vi "adjacent_ttl_parameters.vi"(8 "Deprivation\nparameters":T1={"Frame Row"=0, "Kstd"=40.0, "# Images for\nsleep detection"=10, "Kmean"=1.5, "Start time of sleep detection (images):"=1000, 0, "Length (images)"=3600, "# TTL"=10000, "by x images after first detection"=0, "PauseBetween TTL pulses"=0, "\nby x detections"=9, "# Total immobility\n detections"=0.0, "Pause max # adjacent\nTTL"=0.0, "TTL x start\ntime deprivation\n"=0.0, "Max #\nadjacent TTL"=10000, " Ca2+\nmode"=0} {"?" items=["1", "2", "3", "4"]; "Frame Row" items=["1", "2", "3", "4"]}, 10 "Input \nparameters":T3={"Frame rate (ms)"=2000, "Worm strain"="N2", "Time t"=0, "State"=enum."Image acquisition", "Time elapsed"=0.0, "Max_num_runs"=100000, "#TTL"=0, "Time of start TTL"=100000, "ImSub Value"=0, "Time of last TTL"=0, "Number of Columns"=2, "Number of Rows"=2, "# Adjacent TTL"=0, "Sleep deprivation status"="", "Sleep Detection"=FALSE, "# Sleep detections"=0, "Time of first sleep detection"=0, "Time max # adjacent TTL"=0, "Image t-1"=[], "Image t"=[]} {"Number of Rows" items=["1"=1, "2"=2, "3"=3, "4"=4]; "Number of Columns" items=["1"=1, "2"=2, "3"=3, "4"=4]}) -> (2 "Output \nparameters":T4={"Frame rate (ms)"=2000, "Worm strain"="N2", "Time t"=0, "State"=enum."Image acquisition", "Time elapsed"=0.0, "Max_num_runs"=100000, "#TTL"=0, "Time of start TTL"=100000, "ImSub Value"=0, "Time of last TTL"=0, "Number of Columns"=2, "Number of Rows"=2, "# AdjacentTTL"=0, "Sleep deprivation status"="", "Sleep Detection"=FALSE, "# Sleep detections"=0, "Time of first sleep detection"=0, "Time max # adjacent TTL"=0, "Image t-1"=[], "Image t"=[]} {"Number of Rows" items=["1"=1, "2"=2, "3"=3, "4"=4]; "Number of Columns" items=["1"=1, "2"=2, "3"=3, "4"=4]})   [LabVIEW 2011]
uses:
  state.ctl
panel:
  # "Sleep deprivation settings"
  # "Select deprivation animal"
  # "Row"
  # "Column"
  # "Sleep detection parameters"
  # "Sleep deprivation parameters"
  # "Delay deprivation start:"
  # "Pause deprivation (images):"
  # "Stop deprivation after:"
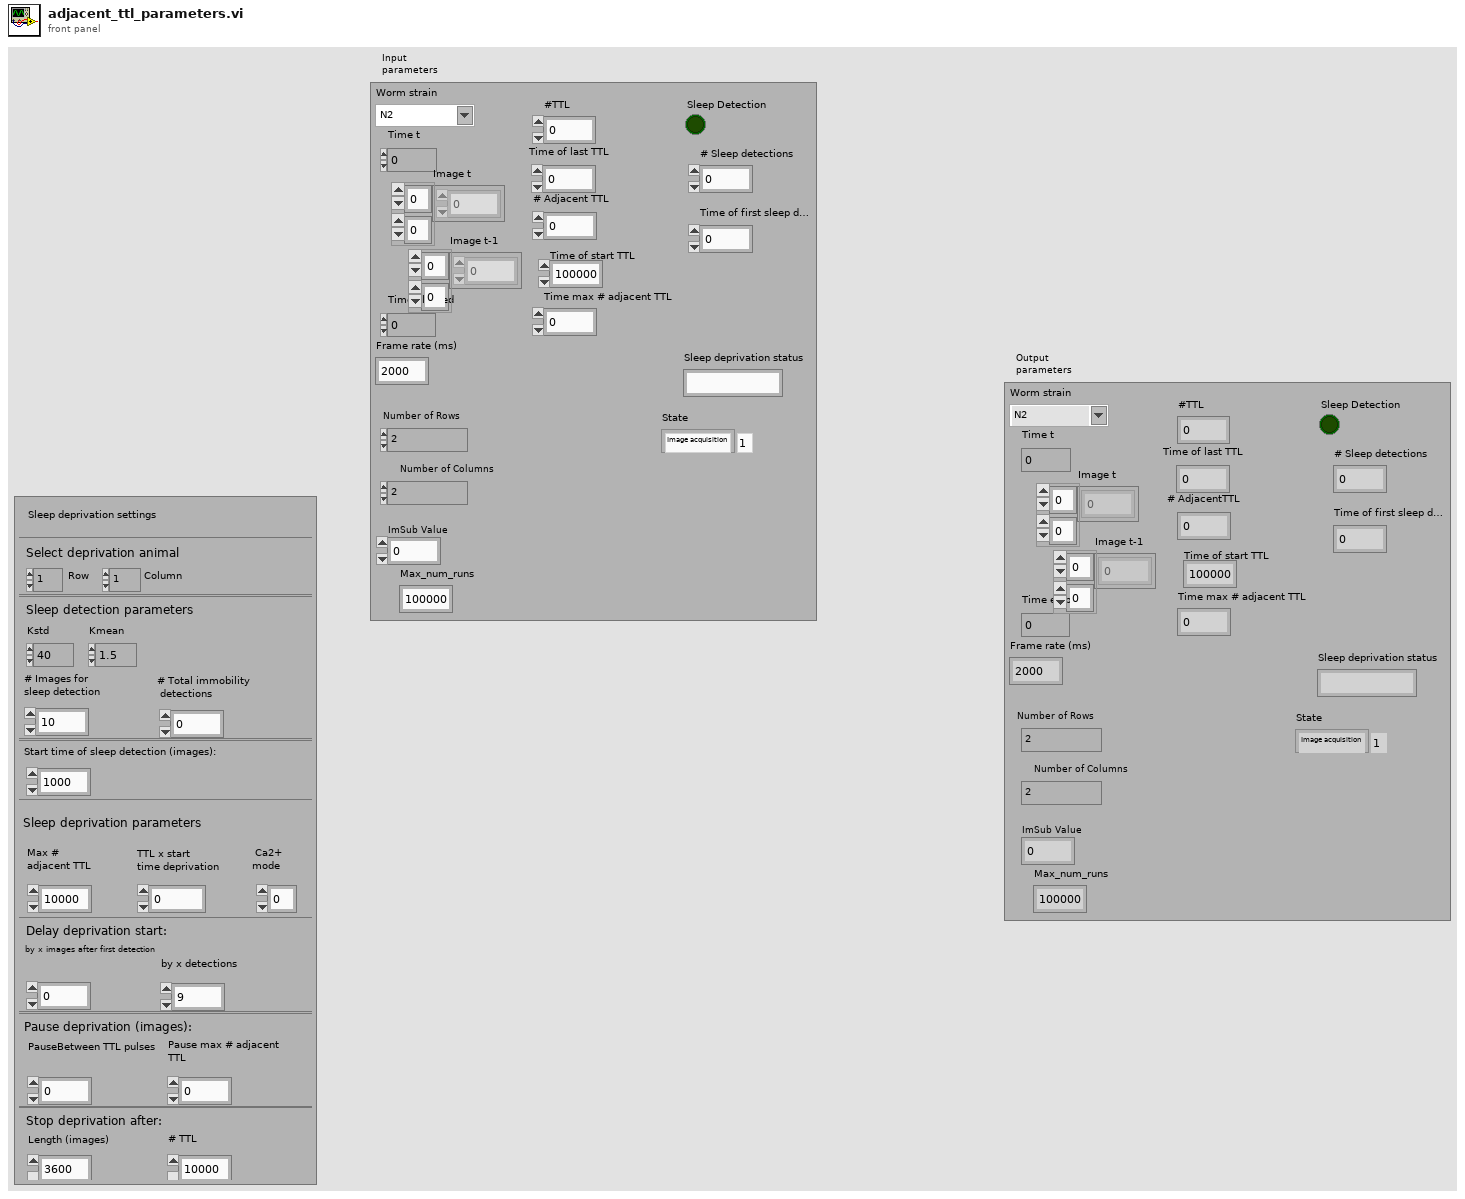
[diagram p1: front panel]
types:
  T1 = cluster{"Frame Row":u32, "Kstd":dbl, "# Images for\nsleep detection":i32, "Kmean":dbl, "Start time of sleep detection (images):":i32, u32, "Length (images)":i32, "# TTL":i32, "by x images after first detection":i32, "PauseBetween TTL pulses":i32, "\nby x detections":i32, "# Total immobility\n detections":dbl, "Pause max # adjacent\nTTL":dbl, "TTL x start\ntime deprivation\n":dbl, "Max #\nadjacent TTL":i32, " Ca2+\nmode":i32}
  T2 = typedef "state.ctl" = enum16{"Initialize measurement", "Image acquisition", "Image processing", "Sleep detection", "Control TTL protocol ", "Sleep deprivation", "Update image & exit condition", "Wait "}
  T3 = cluster{"Frame rate (ms)":u32, "Worm strain":string, "Time t":i32, "State":T2, "Time elapsed":dbl, "Max_num_runs":i32, "#TTL":i32, "Time of start TTL":i32, "ImSub Value":i32, "Time of last TTL":i32, "Number of Columns":u32, "Number of Rows":u32, "# Adjacent TTL":i32, "Sleep deprivation status":string, "Sleep Detection":bool, "# Sleep detections":i32, "Time of first sleep detection":i32, "Time max # adjacent TTL":i32, "Image t-1":i32[][], "Image t":i32[][]}
  T4 = cluster{"Frame rate (ms)":u32, "Worm strain":string, "Time t":i32, "State":T2, "Time elapsed":dbl, "Max_num_runs":i32, "#TTL":i32, "Time of start TTL":i32, "ImSub Value":i32, "Time of last TTL":i32, "Number of Columns":u32, "Number of Rows":u32, "# AdjacentTTL":i32, "Sleep deprivation status":string, "Sleep Detection":bool, "# Sleep detections":i32, "Time of first sleep detection":i32, "Time max # adjacent TTL":i32, "Image t-1":i32[][], "Image t":i32[][]}
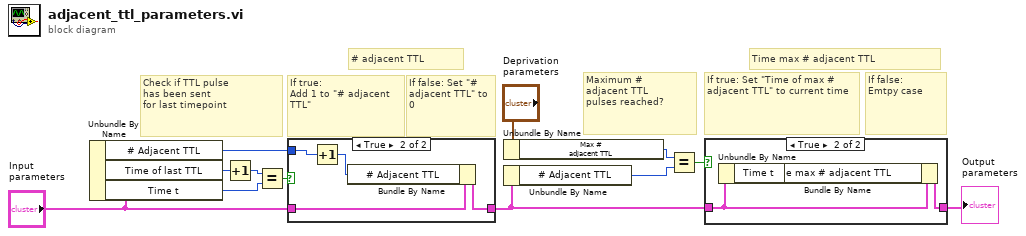
[diagram p0: block diagram]
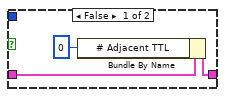
[diagram p2: hidden frame]
diagram:
  # "Maximum # \nadjacent TTL\npulses reached?"
  # "# adjacent TTL"
  # "Check if TTL pulse \nhas been sent \nfor last timepoint"
  # "If false: Set \"# adjacent TTL\" to 0"
  # "If true:\nAdd 1 to \"# adjacent TTL\""
  # "If false: \nEmtpy case"
  # "If true: Set \"Time of max # adjacent TTL\" to current time"
  # "Time max # adjacent TTL"
  n1 = Unbundle By Name("Input \nparameters") -> ("# Adjacent TTL"=w5:i32, "Time of last TTL"=w6:i32, "Time t"=w7:i32)
  n2 = Increment(x=w6) -> (x+1=w8:i32)
  n3 = Equal?(x=w8, y=w7) -> (x = y?=w9:bool)
  n4 = case shown="True" w9 {
    tunnel: "Input \nparameters" -> [w15 w18]
    tunnel: [w14 w19] -> w4
    tunnel: w5 -> [_ w16]
    frame False {
      n5 = Bundle By Name(cluster=w15, "# Adjacent TTL"=0 ("number of adjecentTTL")) -> (w14:T3)
    }
    frame True {
      n6 = Increment(x=w16) -> (x+1=w17:i32)
      n7 = Bundle By Name(cluster=w18, "# Adjacent TTL"=w17) -> (w19:T3)
    }
  }
  n8 = Unbundle By Name("Deprivation\nparameters") -> ("Max #\nadjacent TTL"=w12:i32)
  n9 = Unbundle By Name(w4) -> ("# Adjacent TTL"=w11:i32)
  n10 = Equal?(x=w12, y=w11) -> (x = y?=w10:bool)
  n11 = case shown="True" w10 {
    tunnel: w4 -> [w20 w22]
    tunnel: [w20 w23] -> w2
    frame False {
    }
    frame True {
      n12 = Unbundle By Name(w22) -> ("Time t"=w21:i32)
      n13 = Bundle By Name(cluster=w22, "Time max # adjacent TTL"=w21) -> (w23:T3)
    }
  }
  "Output \nparameters" <- w2
